vi "GetDesktopWindow.vi"(8 "error in (no error)":errorcluster) -> (0 "error out":errorcluster, 3 "hWnd":T1)   [LabVIEW 2011]
doc: "GetDesktopWindow\nThe GetDesktopWindow function returns a handle to the desktop window. The desktop window covers the entire screen. The desktop window is the area on top of which all icons and other windows are painted. \n\nHWND GetDesktopWindow(VOID)\n \nParameters\nThis function has no parameters. \n\nReturn Values\nThe return value is a handle to the desktop window."
uses:
  hWnd.ctl
  user32.dll
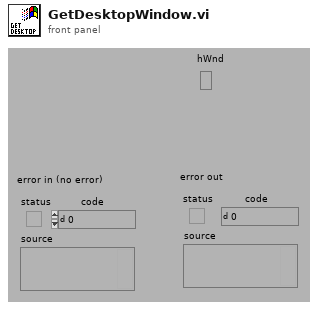
[diagram p1: front panel]
types:
  T1 = typedef "hWnd.ctl" = refnum<k1>
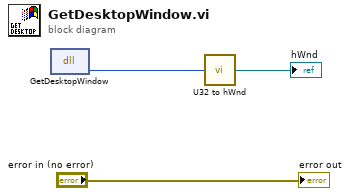
[diagram p0: block diagram]
diagram:
  n1 = dll-call lib="User32.dll" fn="GetDesktopWindow"() -> ("hWndDesktop"=w2:u32)  [unwired: 3 in, 2 out]
  n2 = call "U32 to hWnd.vi"("hWnd"=w2) -> ("hWnd"=→"hWnd":T1)  [unwired: 4 out]
  "error out" <- "error in (no error)"
